vi "main.vi"() -> ()   [LabVIEW 2015, in "example_01.lvlib"]
uses:
  example_01.lvlib
  _controls/recipes.ctl
  _controls/steps_actions.ctl
  <userlib>/antonio-alexander/lv-recipe-machine/public/_controls/configuration.ctl
  _controls/steps_actions_data.ctl
  <userlib>/antonio-alexander/lv-recipe-machine/public/_controls/mode.ctl
  <userlib>/antonio-alexander/lv-recipe-machine/lv-recipe-machine.lvlib
panel:
  out "data":variant
  out "error":errorcluster
  in  "clear_info":bool
  in  "tab_control":enum32{"help", "manual", "automatic"}(tab)
  in  "comparison_value":dbl=0.5 min=0.0 max=1.0
  in  "manual_action":T1=enum."manual_random"
  in  "wait_time_ms":i32=1000
  in  "execute":bool
  out "comparison":bool
  out "random_data":dbl
  out "wait_elapsed_time":dbl format="%<%H:%M:%S%3u>t"
  out "step_elapsed_time":dbl format="%<%H:%M:%S%3u>t"
  out "step_elapsed_time":dbl format="%<%H:%M:%S%3u>t"
  in  "recipe":T2=enum."random_wait"
  out "current iteration":i32
  out "random_data":dbl
  out "recipe_elapsed_time":dbl format="%<%H:%M:%S%3u>t"
  out "wait_elapsed_time":dbl format="%<%H:%M:%S%3u>t"
  in  "start":bool
  in  "pause":bool
  in  "abort":bool
  in  "resume":bool
  in  "iterations":i32=10
  in  "max_value":dbl=0.9
  out "comparison":bool
  in  "stop":bool
  in  "refresh_rate_ms":i32=-1
  out "action_step":string
  out "state":string
  out "mode":string
  # "Changing the tab will programatically change the mode to automatic or manual (going back to help doesn't change the mode). On start the indicators will reset to their defaults, once you execute certain processes the indicators will update as processes happen.\n\nThe refresh_rate_ms can be used to set (or unset) the timeout in ms, to update the status, while the clear errors button can be used to \"unset\" the error, errors will latch. \n\nThe stop button can be used to exit the application as a whole.\n\n\n\n\n-Antonio Alexander"
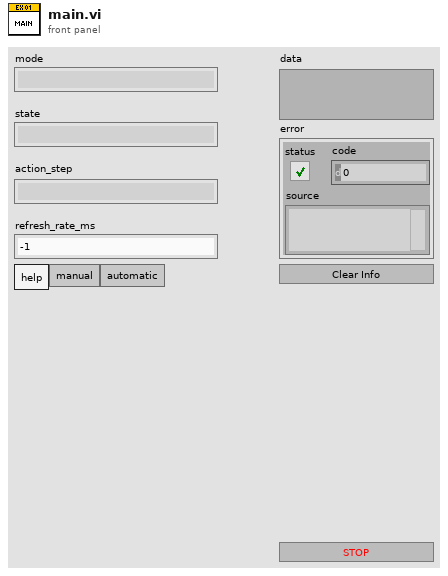
[diagram p1: front panel]
types:
  T1 = typedef "example_01.lvlib/steps_actions.ctl" = enum16{"<steps_actions>", "manual_random", "manual_comparison", "manual_wait", "auto_random", "auto_wait", "criteria_initialize", "criteria_count", "criteria_comparison", "transition_simple", "transition_count", "transition_comparison", "launch_wait", "<null>"}
  T2 = typedef "example_01.lvlib/recipes.ctl" = enum16{"<recipes>", "wait_random", "random_wait", "count", "comparison", "launch", "<null>"}
  T3 = typedef "lv-recipe-machine.lvlib/configuration.ctl" = cluster{dbl}
  T4 = typedef "example_01.lvlib/steps_actions_data.ctl" = cluster{"step_action":T1, "data":variant}
  T5 = typedef "lv-recipe-machine.lvlib/mode.ctl" = enum16{"<mode>", "manual", "automatic", "<null>"}
  T6 = cluster{"change_out":refnum<event-registration>, "status_event_registration":refnum<event-registration>}
  T7 = typedef "lv-recipe-machine.lvlib/status.ctl" = cluster{"mode":T5, "manual_state":T8, "automatic_state":T9, "automatic_data":variant, "step":string, "recipe_elapsed_time":dbl, "step_elapsed_time":dbl, "recipe_error":errorcluster}
  T8 = typedef "lv-recipe-machine.lvlib/manual_state.ctl" = enum16{"<manual_state>", "failed", "action", "running", "idle", "<null>"}
  T9 = typedef "lv-recipe-machine.lvlib/automatic_state.ctl" = enum16{"<automatic_state>", "failed", "idle", "running", "paused", "stopped", "<null>"}
  T10 = typedef "lv-recipe-machine.lvlib/recipe_step.ctl" = cluster{"step":string, "data":variant}
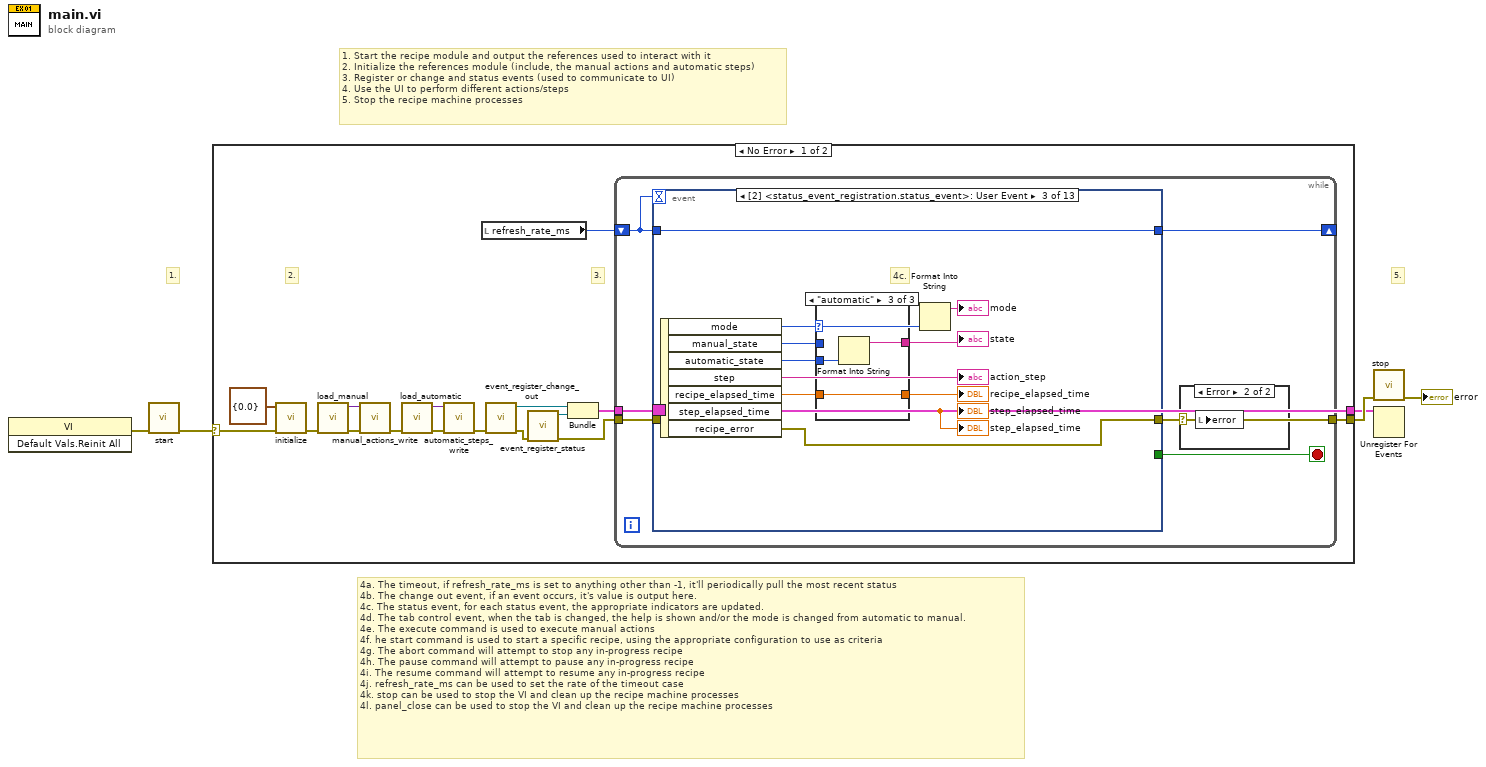
[diagram p0: block diagram]
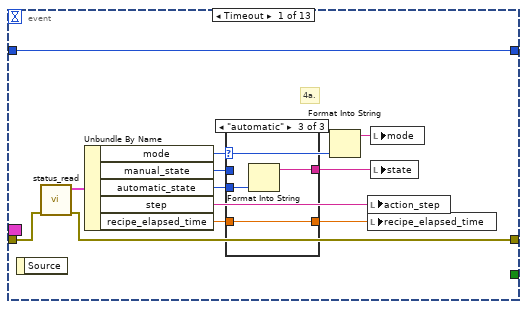
[diagram p3: hidden frame]
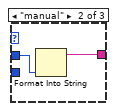
[diagram p5: hidden frame]
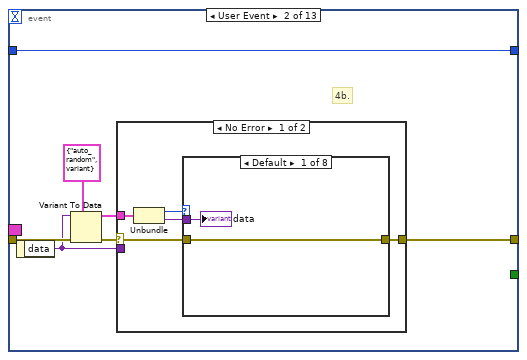
[diagram p6: hidden frame]
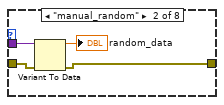
[diagram p7: hidden frame]
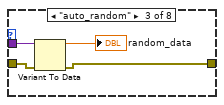
[diagram p8: hidden frame]
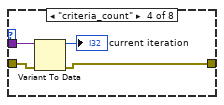
[diagram p9: hidden frame]
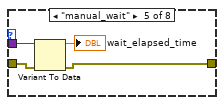
[diagram p10: hidden frame]
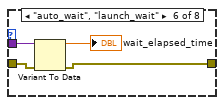
[diagram p11: hidden frame]
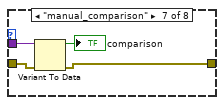
[diagram p12: hidden frame]
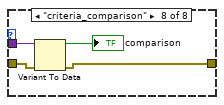
[diagram p13: hidden frame]
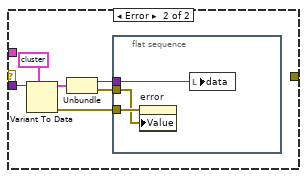
[diagram p14: hidden frame]
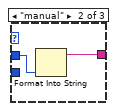
[diagram p16: hidden frame]
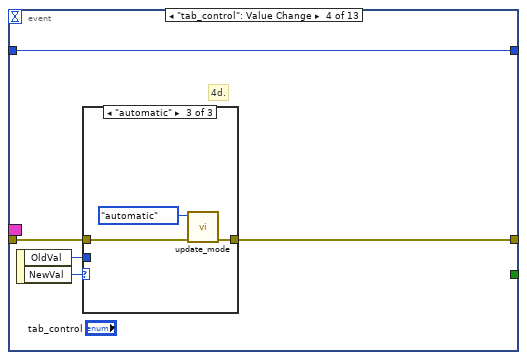
[diagram p17: hidden frame]
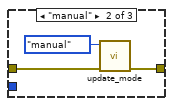
[diagram p19: hidden frame]
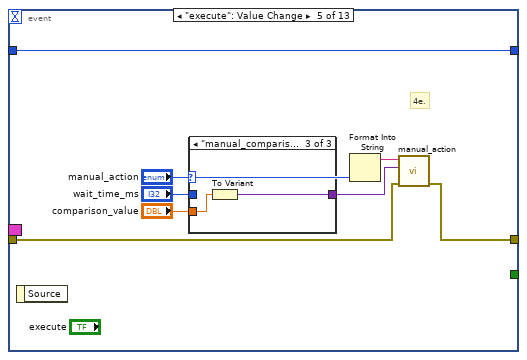
[diagram p20: hidden frame]
diagram:
  # "4a. The timeout, if refresh_rate_ms is set to anything other than -1, it'll periodically pull the most recent status\n4b. The change out event, if an event occurs, it's value is output here. \n4c. The status event, for each status event, the appropriate indicators are updated.\n4d. The tab control event, when the tab is changed, the help is shown and/or the mode is changed from automatic to manual.\n4e. The execute command is used to execute manual actions \n4f. he start command is used to start a specific recipe, using the appropriate configuration to use as criteria\n4g. The abort command will attempt to stop any in-progress recipe \n4h. The pause command will attempt to pause any in-progress recipe \n4i. The resume command will attempt to resume any in-progress recipe\n4j. refresh_rate_ms can be used to set the rate of the timeout case\n4k. stop can be used to stop the VI and clean up the recipe machine processes\n4l. panel_close can be used to stop the VI and clean up the recipe machine processes"
  # "5."
  # "1. Start the recipe module and output the references used to interact with it\n2. Initialize the references module (include, the manual actions and automatic steps)\n3. Register or change and status events (used to communicate to UI)\n4. Use the UI to perform different actions/steps\n5. Stop the recipe machine processes"
  # "1."
  n1 = invoke class="VI" method="Default Vals.Reinit All"() -> (error out=w1:errorcluster)  [unwired: 3 in, 2 out]
  n2 = call <userlib>:"start.vi"("error in (no error)"=w1) -> ("error out"=w3:errorcluster)  [unwired: 10 in]
  n3 = case shown="No Error" w3 {
    selector: w3 -> [w19 w184]
    tunnel: [w21 w184] -> w5
    tunnel: [w7 _] -> w4
    frame No Error {
      # "3."
      # "2."
      n4 = call <userlib>:"initialize.vi"("error in (no error)"=w19, "configuration"=T3 {0.0}) -> ("error out"=w14:errorcluster)  [unwired: 9 in]
      n5 = call "load_manual.vi"("error in (no error)"=w14) -> ("error out"=w17:errorcluster, "manual_actions out"=w13:variant)  [unwired: 8 in, 1 out]
      n6 = call <userlib>:"manual_actions_write.vi"("error in (no error)"=w17, "manual_actions"=w13) -> ("error out"=w16:errorcluster)  [unwired: 8 in, 1 out]
      n7 = call "load_automatic.vi"("error in (no error)"=w16) -> ("error out"=w15:errorcluster, "automatic_steps out"=w12:variant)  [unwired: 8 in, 1 out]
      n8 = call <userlib>:"automatic_steps_write.vi"("error in (no error)"=w15, "automatic_steps"=w12) -> ("error out"=w9:errorcluster)  [unwired: 8 in, 1 out]
      n9 = local read "refresh_rate_ms"() -> (w20:i32)
      n10 = call <userlib>:"event_register_change_out.vi"("error in (no error)"=w9) -> ("error out"=w8:errorcluster, "change_out"=w11:refnum<event-registration>)  [unwired: 9 in]
      n11 = call <userlib>:"event_register_status.vi"("error in (no error)"=w8) -> ("error out"=w6:errorcluster, "status_event_registration"=w10:refnum<event-registration>)  [unwired: 9 in]
      n12 = Bundle("change_out"=w11, "status_event_registration"=w10) -> (w7:T6)  [unwired: 1 in]
      n13 = while {
        tunnel: w6 -> [w27]
        tunnel: [w24] -> w21
        tunnel: w7 -> [w25]
        shift-right: [w23] -> _
        shift-left: w20 -> [w22]
        stop <- w26 stop-if-true
        n14 = event shown="[2] <status_event_registration.status_event>: User Event" {
          selector: w25 -> [_ _ _ _ _ _ _ _ _ _ _ _ _]
          dyn-events: _ -> [_ _ _ _ _ _ _ _ _ _ _ _ _]
          timeout: w22 -> [_ _ _ _ _ _ _ _ _ _ _ _ _]
          tunnel: w27 -> [w40 w52 _ w115 w132 w148 w164 w167 w170 _ w174 w177 w182]
          tunnel: [w39 w51 w97 w114 w130 w141 w163 w166 w169 _ w172 w176 w181] -> w24
          tunnel: [_ _ _ _ _ _ _ _ _ _ _ TRUE w180] -> w26
          tunnel: w22 -> [w31 w50 w102 w117 w126 w144 w162 w165 w168 _ w175 w178 w183]
          tunnel: [w31 w50 w102 w117 w126 w144 w162 w165 w168 "refresh_rate_ms" w175 w178 w183] -> w23
          event Timeout {
            # "4a."
            n15 = event-data() -> ()  [unwired: 1 in, 1 out]
            n16 = call <userlib>:"status_read.vi"("error in (no error)"=w40) -> ("error out"=w39:errorcluster, "status"=w38:T7)  [unwired: 9 in]
            n17 = Unbundle By Name(w38) -> ("mode"=w35:T5, "manual_state"=w37:T8, "automatic_state"=w36:T9, "step"=w32:string, "recipe_elapsed_time"=w30:dbl)
            n18 = case shown="\"automatic\"" w35 {
              tunnel: w37 -> [_ w42 _]
              tunnel: w36 -> [_ _ w44]
              tunnel: [_ w41 w45] -> w33
              tunnel: w30 -> [_ _ w43]
              tunnel: [_ _ w43] -> w29
              frame Default {
              }
              frame "manual" {
                n19 = Format Into String(w42) -> (resulting string=w41:string)  [unwired: 3 in, 1 out]
              }
              frame "automatic" {
                n20 = Format Into String(w44) -> (resulting string=w45:string)  [unwired: 3 in, 1 out]
              }
            }
            n21 = Format Into String(w35) -> (resulting string=w34:string)  [unwired: 3 in, 1 out]
            n22 = local write "action_step"(w32) -> ()
            n23 = local write "recipe_elapsed_time"(w29) -> ()
            n24 = local write "mode"(w34) -> ()
            n25 = local write "state"(w33) -> ()
          }
          event User Event {
            # "4b."
            n26 = event-data() -> ("data"=w46:variant)  [unwired: 1 in]
            n27 = Variant To Data(error in=w52, type=T4 {"step_action"=enum."auto_random", "data"=variant}, Variant=w46) -> (data=w48:T4, error out=w47:errorcluster)
            n28 = case shown="No Error" w47 {
              selector: w47 -> [w55 _]
              tunnel: [w57 _] -> w51
              tunnel: w48 -> [w56 _]
              tunnel: w46 -> [_ w93]
              frame No Error {
                n29 = Unbundle(w56) -> ("step_action"=w53:T1, "data"=w54:variant)
                n30 = case shown="Default" w53 {
                  tunnel: w55 -> [w59 w63 w67 w71 w75 w79 w83 w87]
                  tunnel: [w59 w60 w65 w68 w73 w77 w81 w85] -> w57
                  tunnel: w54 -> [w58 w62 w66 w70 w74 w78 w82 w86]
                  frame Default {
                    "data" <- w58
                  }
                  frame "manual_random" {
                    n31 = Variant To Data(error in=w63, Variant=w62) -> (data=→"random_data":dbl, error out=w60:errorcluster)  [unwired: 1 in]
                  }
                  frame "auto_random" {
                    n32 = Variant To Data(error in=w67, Variant=w66) -> (data=→"random_data":dbl, error out=w65:errorcluster)  [unwired: 1 in]
                  }
                  frame "criteria_count" {
                    n33 = Variant To Data(error in=w71, Variant=w70) -> (data=→"current iteration":i32, error out=w68:errorcluster)  [unwired: 1 in]
                  }
                  frame "manual_wait" {
                    n34 = Variant To Data(error in=w75, Variant=w74) -> (data=→"wait_elapsed_time":dbl, error out=w73:errorcluster)  [unwired: 1 in]
                  }
                  frame "auto_wait", "launch_wait" {
                    n35 = Variant To Data(error in=w79, Variant=w78) -> (data=→"wait_elapsed_time":dbl, error out=w77:errorcluster)  [unwired: 1 in]
                  }
                  frame "manual_comparison" {
                    n36 = Variant To Data(error in=w83, Variant=w82) -> (data=→"comparison":bool, error out=w81:errorcluster)  [unwired: 1 in]
                  }
                  frame "criteria_comparison" {
                    n37 = Variant To Data(error in=w87, Variant=w86) -> (data=→"comparison":bool, error out=w85:errorcluster)  [unwired: 1 in]
                  }
                }
              }
              frame Error {
                n38 = Variant To Data(type=cluster{variant, "error constant":errorcluster} {variant, "error constant"={"status"=FALSE, "code"=0, "source"=""}}, Variant=w93) -> (data=w92:cluster{variant, "error constant":errorcluster}, error out=w88:errorcluster)  [unwired: 1 in]
                n39 = Unbundle(w92) -> (w90:variant, "error constant"=w89:errorcluster)
                n40 = flat-sequence {
                  tunnel: w90 -> [w94]
                  tunnel: w89 -> [w95]
                  tunnel: w88 -> [w96]
                  frame #0 {
                    n41 = property on="error" class="Clust (strict)"(error in=w96, "Value"=w95) -> ()  [unwired: 1 in, 2 out]
                    n42 = local write "data"(w94) -> ()
                  }
                }
              }
            }
          }
          event User Event {
            # "4c."
            n43 = event-data() -> ("mode"=w104:T5, "manual_state"=w107:T8, "automatic_state"=w106:T9, "step"=→"action_step":string, "recipe_elapsed_time"=w100:dbl, "step_elapsed_time"=→"step_elapsed_time" →"step_elapsed_time":dbl, "recipe_error"=w97:errorcluster)  [unwired: 1 in]
            n44 = case shown="\"automatic\"" w104 {
              tunnel: w107 -> [_ w108 _]
              tunnel: w106 -> [_ _ w111]
              tunnel: [_ w109 w112] -> w105
              tunnel: w100 -> [_ _ w110]
              tunnel: [_ _ w110] -> w99
              frame Default {
              }
              frame "manual" {
                n45 = Format Into String(w108) -> (resulting string=w109:string)  [unwired: 3 in, 1 out]
              }
              frame "automatic" {
                n46 = Format Into String(w111) -> (resulting string=w112:string)  [unwired: 3 in, 1 out]
              }
            }
            "state" <- w105
            "recipe_elapsed_time" <- w99
            n47 = Format Into String(w104) -> (resulting string=→"mode":string)  [unwired: 3 in, 1 out]
          }
          event "tab_control": Value Change {
            # "4d."
            n48 = event-data() -> ("OldVal"=w113:enum32{"help", "manual", "automatic"}, "NewVal"=w116:enum32{"help", "manual", "automatic"})  [unwired: 1 in]
            n49 = case shown="\"automatic\"" w116 {
              tunnel: w115 -> [w118 w120 w123]
              tunnel: [w118 w119 w122] -> w114
              tunnel: w113 -> [_ _ _]
              frame Default {
              }
              frame "manual" {
                n50 = call <userlib>:"update_mode.vi"("error in (no error)"=w120, "mode"=mode."manual") -> ("error out"=w119:errorcluster)  [unwired: 9 in]
              }
              frame "automatic" {
                n51 = call <userlib>:"update_mode.vi"("error in (no error)"=w123, "mode"=mode."automatic") -> ("error out"=w122:errorcluster)  [unwired: 9 in]
              }
            }
          }
          event "execute": Value Change {
            # "4e."
            n52 = event-data() -> ()  [unwired: 1 in, 1 out]
            n53 = case shown="\"manual_comparison\"" "manual_action" {
              tunnel: "wait_time_ms" -> [_ w134 _]
              tunnel: [_ w133 w136] -> w127
              tunnel: "comparison_value" -> [_ _ w135]
              frame Default {
              }
              frame "manual_wait" {
                n54 = To Variant(anything=w134) -> (Variant=w133:variant)
              }
              frame "manual_comparison" {
                n55 = To Variant(anything=w135) -> (Variant=w136:variant)
              }
            }
            n56 = Format Into String("manual_action") -> (resulting string=w131:string)  [unwired: 3 in, 1 out]
            n57 = call <userlib>:"manual_action.vi"("error in (no error)"=w132, "data"=w127, "step"=w131) -> ("error out"=w130:errorcluster)  [unwired: 8 in]
          }
          event "start": Value Change {
            # "4f."
            n58 = event-data() -> ()  [unwired: 1 in, 1 out]
            n59 = call "load_recipes.vi"("error in (no error)"=w148, "recipe"="recipe") -> ("error out"=w146:errorcluster, "transition []"=w143:string, "recipe []"=w147:T10[])  [unwired: 7 in]
            n60 = call <userlib>:"automatic_recipe_write.vi"("error in (no error)"=w146, "transition"=w143, "recipe []"=w147) -> ("error out"=w145:errorcluster)  [unwired: 8 in]
            n61 = case shown="\"comparison\"" "recipe" {
              selector: "recipe" -> [_ w153 w159]
              tunnel: w145 -> [w149 w155 w161]
              tunnel: [w149 w155 w161] -> w140
              tunnel: "iterations" -> [_ w152 _]
              tunnel: "max_value" -> [_ _ w158]
              tunnel: [_ w154 w160] -> w137
              frame Default {
              }
              frame "count" {
                n62 = To Variant(anything=w152) -> (Variant=w150:variant)
                n63 = Bundle("recipe"=w153, "Variant"=w150) -> (w151:cluster{"recipe":T2, "Variant":variant})  [unwired: 1 in]
                n64 = To Variant(anything=w151) -> (Variant=w154:variant)
              }
              frame "comparison" {
                n65 = To Variant(anything=w158) -> (Variant=w156:variant)
                n66 = Bundle("recipe"=w159, "Variant"=w156) -> (w157:cluster{"recipe":T2, "Variant":variant})  [unwired: 1 in]
                n67 = To Variant(anything=w157) -> (Variant=w160:variant)
              }
            }
            n68 = call <userlib>:"automatic_start.vi"("error in (no error)"=w140, "criteria"=w137) -> ("error out"=w141:errorcluster)  [unwired: 9 in]
          }
          event "abort": Value Change {
            # "4g."
            n69 = event-data() -> ()  [unwired: 1 in, 1 out]
            n70 = call <userlib>:"automatic_abort.vi"("error in (no error)"=w164) -> ("error out"=w163:errorcluster)  [unwired: 10 in]
          }
          event "pause": Value Change {
            # "4h."
            n71 = event-data() -> ()  [unwired: 1 in, 1 out]
            n72 = call <userlib>:"automatic_pause.vi"("error in (no error)"=w167) -> ("error out"=w166:errorcluster)  [unwired: 10 in]
          }
          event "resume": Value Change {
            # "4i."
            n73 = event-data() -> ()  [unwired: 1 in, 1 out]
            n74 = call <userlib>:"automatic_resume.vi"("error in (no error)"=w170) -> ("error out"=w169:errorcluster)  [unwired: 10 in]
          }
          event "refresh_rate_ms": Value Change {
            # "4j."
            n75 = event-data() -> ()  [unwired: 1 in, 1 out]
          }
          event "clear_info": Value Change {
            n76 = event-data() -> ()  [unwired: 1 in, 1 out]
            n77 = invoke on="error" class="Clust (strict)" method="Reinit To Default"(error in=w174) -> (error out=w173:errorcluster)  [unwired: 2 in, 2 out]
            n78 = invoke on="data" class="LVVar" method="Reinit To Default"(error in=w173) -> (error out=w172:errorcluster)  [unwired: 2 in, 2 out]
          }
          event "stop": Value Change {
            # "4k."
            n79 = event-data() -> ()  [unwired: 1 in, 1 out]
            n80 = call <userlib>:"shutdown.vi"("error in (no error)"=w177) -> ("error out"=w176:errorcluster)  [unwired: 10 in]
          }
          event Panel Close? {
            w180 = TRUE
            # "4l."
            n81 = event-data() -> ()  [unwired: 1 in, 1 out]
            n82 = call <userlib>:"shutdown.vi"("error in (no error)"=w182) -> ("error out"=w181:errorcluster)  [unwired: 10 in]
            n83 = event-data("Discard?"=w180) -> ()  [unwired: 1 in, 1 out]
          }
        }
        n84 = case shown="Error" w24 {
          selector: w24 -> [_ w28]
          frame No Error {
          }
          frame Error {
            n85 = local write "error"(w28) -> ()
          }
        }
      }
    }
    frame Error {
    }
  }
  n86 = call <userlib>:"stop.vi"("error in (no error)"=w5) -> ("error out"=→"error":errorcluster)  [unwired: 10 in]
  n87 = Unregister For Events(event registration refnum=w4) -> ()  [unwired: 1 in, 1 out]
